vi "Speed ControlBeforeNetwork.vi"() -> ()   [LabVIEW 2014]
uses:
  C:/Users/Sam/OneDrive/Project/Software/MyRIO Software/MyTypeDefs/EncoderController.ctl
  <vilib>/Platform/TimedLoop/XDataNode/timing_clust.ctl
  <vilib>/Platform/TimedLoop/XDataNode/nitl_modes.ctl
  <vilib>/Platform/TimedLoop/XDataNode/wakeup.ctl
  <vilib>/Platform/TimedLoop/XDataNode/loadnilvce.vi
  <vilib>/addons/control/pid/pid.llb/PID (DBL).vi
  <vilib>/addons/control/pid/pid.llb/PID Percentage to EGU (DBL).vi
  <vilib>/platform/TimedLoop/XDataNode/XDataNode.xnode
  <vilib>/addons/control/pid/NI_PID_pid.lvlib
  <vilib>/Platform/TimedLoop/XDataNode/XDNodeRunTimeDep.lvlib
panel:
  out "output (EGU)":dbl format="%.2f"
  in  "Encoder 4 Controller":T1={"Sample time (uS)"=300000, "Reset"=FALSE}
  out "Current Speed":dbl(graph)
  out "PID output":dbl(graph)
  out "Current Speed RPM":dbl
  in  "Stop Button":bool
  in  "PID gains":T2={"proportional gain (Kc)"=0.6, "integral time (Ti, min)"=0.01, "derivative time (Td, min)"=0.0} {"derivative time (Td, min)" format="%.3f"; "integral time (Ti, min)" format="%.3f"; "proportional gain (Kc)" format="%.3f"}
  in  "Setpoint Speed (RPM)":dbl=1.0 format="%.2f"
  # "0.8, 0. 0 is stable but theres a large offset\nsystem is slow to settle, increase Ti"
  # "Kp=2.04, Ti=0.15, Td=0.0375"
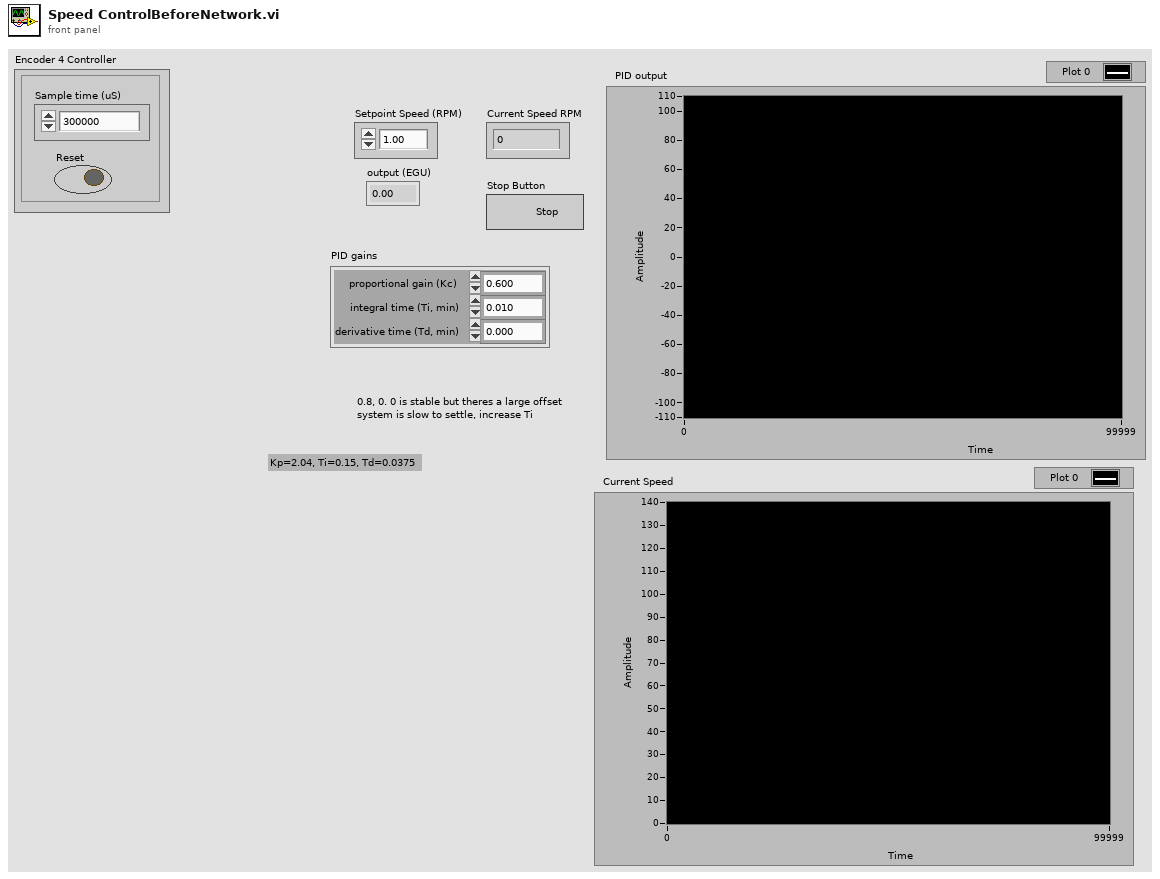
[diagram p1: front panel]
types:
  T1 = typedef "EncoderController.ctl" = cluster{"Sample time (uS)":u32, "Reset":bool}
  T2 = cluster{"proportional gain (Kc)":dbl, "integral time (Ti, min)":dbl, "derivative time (Td, min)":dbl}
  T3 = cluster{bool, "Tick Count(uSec)":u32, "Counter Value":i32, "x-y":i32}
  T4 = typedef "XDNodeRunTimeDep.lvlib/timing_clust.ctl" = cluster{"Expected End [f-1]":u64, "Actual End [f-1]":u64, "Finished Late? [f-1]":bool, "Expected End [i-1]":u64, "Actual End [i-1]":u64, "Finished Late? [i-1]":bool, "Expected Start [i]":u64, "Actual Start [i]":u64, "Expected Start [f]":u64, "Actual Start [f]":u64, "Source Name":string, "Structure Name":string, "Period":i64, "Deadline":i64, "Offset":i64, "Start":i64, "Priority":i32, "Timeout":i32, "Mode":T5, "Wakeup Reason":T6, "Error":errorcluster, "Source Type":string, "Secondary Source Type":string, "Global End Time":u64, "Global Start Time":u64, "Frame Duration":u64, "Iteration Duration":u64, "Assigned CPU":i32, "I/O Scan Engine Mode":u32}
  T5 = typedef "XDNodeRunTimeDep.lvlib/nitl_modes.ctl" = enum32{"No Change", "Process missed periods, maintain original phase", "Discard missed periods, maintain original phase", "Process missed periods, ignore original phase", "Discard missed periods, ignore original phase"}
  T6 = typedef "XDNodeRunTimeDep.lvlib/wakeup.ctl" = enum32{"Normal", "Aborted", "Asynchronous wakeup", "Timing source error", "Timed loop error", "Timeout"}
  T7 = typedef "EncoderIndicator.ctl" = cluster{"Position":dbl, "Velocity RPM":dbl, "Velocity RPS":dbl}
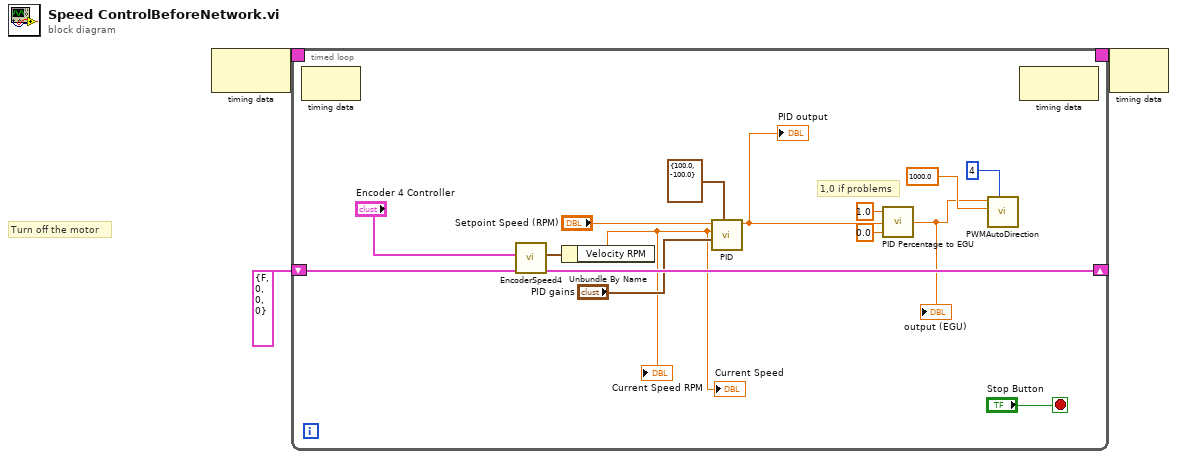
[diagram p0: block diagram]
diagram:
  # "Turn off the motor"
  n1 = node-c288() -> (w2:T4)  [unwired: 1 in]
  n2 = timed-loop {
    shift-right: [w17] -> _
    shift-left: T3 {FALSE, "Tick Count(uSec)"=0, "Counter Value"=0, "x-y"=0} ("Cluster out") -> [w18]
    timing: w2 -> [_]
    timing-out: [_] -> w1
    stop <- "Stop Button" stop-if-true
    # "1,0 if problems"
    n3 = node-c288() -> ()  [unwired: 1 in, 1 out]
    n4 = call "EncoderSpeed4.vi"("Cluster in"=w18, "Encoder 4 Controller"="Encoder 4 Controller") -> ("Cluster out"=w17:T3, "Encoder 4 Indicator"=w16:T7)  [unwired: 7 in, 1 out]
    n5 = Unbundle By Name(w16) -> ("Velocity RPM"=w12:dbl)
    "Current Speed RPM" <- w12
    "Current Speed" <- w12
    n6 = call-poly <vilib>:"PID.vi"("output range"=cluster{"output high":dbl, "output low":dbl} {"output high"=100.0, "output low"=-100.0}, "PID gains"="PID gains", "process variable"=w12, "setpoint"="Setpoint Speed (RPM)") -> ("output"=w5:dbl)  [unwired: 6 in, 1 out]
    "PID output" <- w5
    n7 = call-poly <vilib>:"PID Percentage to EGU.vi"("minimum (EGU)"=0.0, "% span"=w5, "maximum (EGU)"=1.0) -> ("output (EGU)"=w6:dbl)  [unwired: 1 in]
    "output (EGU)" <- w6
    n8 = call "PWMAutoDirection.vi"("Motor Select"=i8 4, "PWM Frequency"=1000.0, "DutyCycle"=w6) -> ()  [unwired: 8 in, 1 out]
    n9 = node-c288() -> ()  [unwired: 1 in, 1 out]
  }
  n10 = node-c288(w1) -> ()  [unwired: 1 out]
